vi "Read.vi"(8 "Error In":errorcluster, 11 "PS4 Controller Ref":T3) -> (0 "Error Out":errorcluster, 1 "All Axis":T1, 2 "Buttons":T4, 3 "PS4 Controller Ref":T3)   [LabVIEW 2011, in "LMH-PS4.lvlib"]
doc: "Read the current state of the PS4 controller."
uses:
  LMH-PS4.lvlib
  Private/Type Defs/PS4 Controller Ref.ctl
  Private/Type Defs/Buttons.ctl
  Private/Type Defs/Axis.ctl
  Private/Type Defs/Indicators/DPad Enum.ctl
  <vilib>/Utility/inputDevices.llb/joystickAcquire.vi
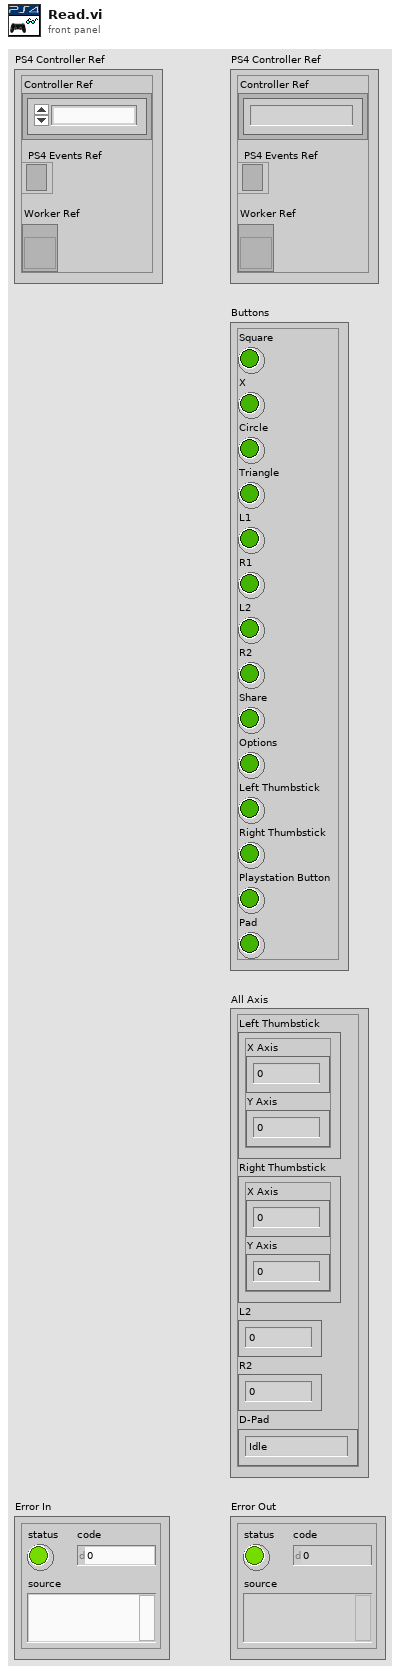
[diagram p1: front panel]
types:
  T1 = typedef "LMH-PS4.lvlib/Axis.ctl" = cluster{"Left Thumbstick":cluster{"X Axis":i32, "Y Axis":i32}, "Right Thumbstick":cluster{"X Axis":i32, "Y Axis":i32}, "L2":i32, "R2":i32, "D-Pad":T2}
  T2 = typedef "LMH-PS4.lvlib/DPad Enum.ctl" = enum16{"Idle", "Up", "Up / Right", "Right", "Down / Right", "Down", "Down / Left", "Left", "Up / Left"}
  T3 = typedef "LMH-PS4.lvlib/PS4 Controller Ref.ctl" = cluster{"Controller Ref":refnum<k1>, "PS4 Events Ref":refnum<event-registration>, "Worker Ref":refnum<vi>}
  T4 = typedef "LMH-PS4.lvlib/Buttons.ctl" = cluster{"Square":bool, "X":bool, "Circle":bool, "Triangle":bool, "L1":bool, "R1":bool, "L2":bool, "R2":bool, "Share":bool, "Options":bool, "Left Thumbstick":bool, "Right Thumbstick":bool, "Playstation Button":bool, "Pad":bool}
  T5 = cluster{"X axis":i32, "Y axis":i32, "Z axis":i32, "X axis rotation":i32, "Y axis rotation":i32, "Z axis rotation":i32, "U axis":i32, "V axis":i32}
  T6 = cluster{"button 1":bool, "button 2":bool, "button 3":bool, "button 4":bool, "button 5":bool, "button 6":bool, "button 7":bool, "button 8":bool, "button 9":bool, "button 10":bool, "button 11":bool, "button 12":bool, "button 13":bool, "button 14":bool, "button 15":bool, "button 16":bool, "button 17":bool, "button 18":bool, "button 19":bool, "button 20":bool, "button 21":bool, "button 22":bool, "button 23":bool, "button 24":bool, "button 25":bool, "button 26":bool, "button 27":bool, "button 28":bool, "button 29":bool, "button 30":bool, "button 31":bool, "button 32":bool}
  T7 = cluster{"pov 1":i32, "pov 2":i32, "pov 3":i32, "pov 4":i32}
  T8 = typedef "DpadEnum.ctl" = enum16{"Idle", "Up", "Up / Right", "Right", "Down / Right", "Down", "Down / Left", "Left", "Up / Left"}
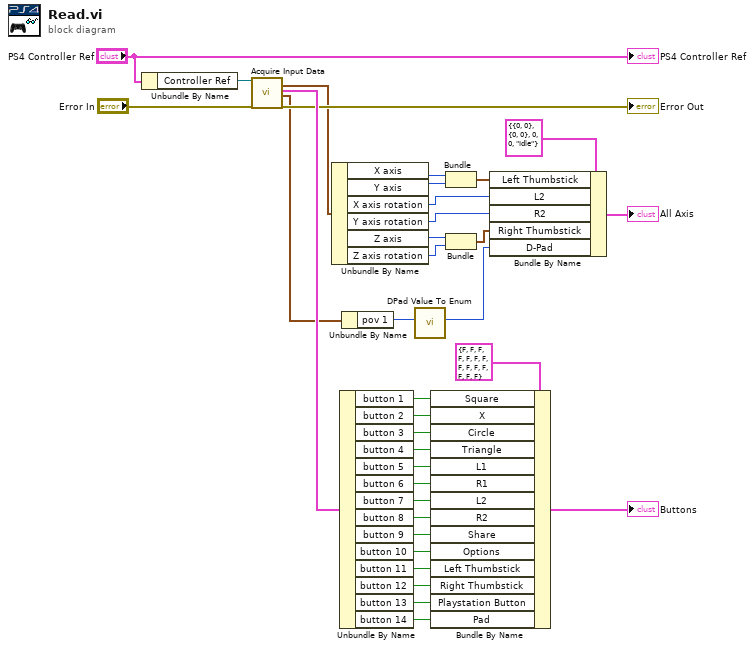
[diagram p0: block diagram]
diagram:
  n1 = Unbundle By Name("PS4 Controller Ref") -> ("Controller Ref"=w35:refnum<k1>)
  n2 = call-poly <vilib>:"Acquire Input Data.vi"("device ID"=w35, "error in (no error)"="Error In") -> ("axis info"=w21:T5, "button info"=w33:T6, "direction info"=w17:T7, "error out"=→"Error Out":errorcluster)  [unwired: 13 in, 1 out]
  n3 = Unbundle By Name(w21) -> ("X axis"=w19:i32, "Y axis"=w20:i32, "X axis rotation"=w7:i32, "Y axis rotation"=w6:i32, "Z axis"=w5:i32, "Z axis rotation"=w4:i32)
  n4 = Unbundle By Name(w33) -> ("button 1"=w31:bool, "button 2"=w30:bool, "button 3"=w29:bool, "button 4"=w28:bool, "button 5"=w27:bool, "button 6"=w26:bool, "button 7"=w25:bool, "button 8"=w24:bool, "button 9"=w23:bool, "button 10"=w22:bool, "button 11"=w13:bool, "button 12"=w12:bool, "button 13"=w11:bool, "button 14"=w10:bool)
  n5 = Unbundle By Name(w17) -> ("pov 1"=w9:i32)
  n6 = call "DPad Value To Enum.vi"("D-Pad Value"=w9) -> ("D-Pad"=w2:T8)  [unwired: 10 in]
  n7 = Bundle By Name(cluster=T4 {"Square"=FALSE, "X"=FALSE, "Circle"=FALSE, "Triangle"=FALSE, "L1"=FALSE, "R1"=FALSE, "L2"=FALSE, "R2"=FALSE, "Share"=FALSE, "Options"=FALSE, "Left Thumbstick"=FALSE, "Right Thumbstick"=FALSE, "Playstation Button"=FALSE, "Pad"=FALSE} ("Buttons"), "Square"=w31, "X"=w30, "Circle"=w29, "Triangle"=w28, "L1"=w27, "R1"=w26, "L2"=w25, "R2"=w24, "Share"=w23, "Options"=w22, "Left Thumbstick"=w13, "Right Thumbstick"=w12, "Playstation Button"=w11, "Pad"=w10) -> (→"Buttons":T4)
  n8 = Bundle("X axis"=w19, "Y axis"=w20) -> (w18:cluster{"X axis":i32, "Y axis":i32})  [unwired: 1 in]
  n9 = Bundle("Z axis"=w5, "Z axis rotation"=w4) -> (w3:cluster{"Z axis":i32, "Z axis rotation":i32})  [unwired: 1 in]
  n10 = Bundle By Name(cluster=T1 {"Left Thumbstick"={"X Axis"=0, "Y Axis"=0}, "Right Thumbstick"={"X Axis"=0, "Y Axis"=0}, "L2"=0, "R2"=0, "D-Pad"=enum."Idle"} ("Axis"), "Left Thumbstick"=w18, "L2"=w7, "R2"=w6, "Right Thumbstick"=w3, "D-Pad"=w2) -> (→"All Axis":T1)
  "PS4 Controller Ref" <- "PS4 Controller Ref"
